vi "Read Users file (popup).vi"(0 "file path (use dialog)":path, 11 "error in (no error)":errorcluster) -> (15 "error out":errorcluster)   [LabVIEW 2012]
doc: "Demo for Type Sensitive Popup\n\nType Sensitive Popup \nCopyright © 2007, J. David Saunders\nAll rights reserved."
uses:
  Desktop/PFC/TypeSensitivePopup_V1_0_1/SubVIs/TSPopup.Popup Cluster.ctl
  Desktop/PFC/TypeSensitivePopup_V1_0_1/SubVIs/TSPopup.Grid.Cell Info.ctl
  Desktop/PFC/TypeSensitivePopup_V1_0_1/SubVIs/TSPopup.Data Type.ctl
  Desktop/PFC/TypeSensitivePopup_V1_0_1/SubVIs/TSPopup.Popup Call Parameters.ctl
  type def/Hyde&Show.ctl
panel:
  out "Info accounts 2":bool
  out "Info pass not secure":bool
  out "Info Dupliclate user":bool
  out "Duplicate user":string[][](table)
  out "Password not secure":string[][](table)
  out "Info accounts":bool
  in  "Cuenta":bool
  in  "Clave":bool
  in  "Name":bool
  in  "Reload":bool
  in  "Save":bool
  in  "Check changes":bool
  in  "Delete":bool
  in  "Show Popup (type only)":T1
  in  "Popups":T3 {"Boolean" items=["False", "True"]; "Ring" items=["None", "User", "Admin"]}
  in  "Cell Info (type only)":T4
  in  "Cancel":bool
  in  "?":string[][](table)
  # "Type Sensitive\nPopup"
  # "Boolean Colors"
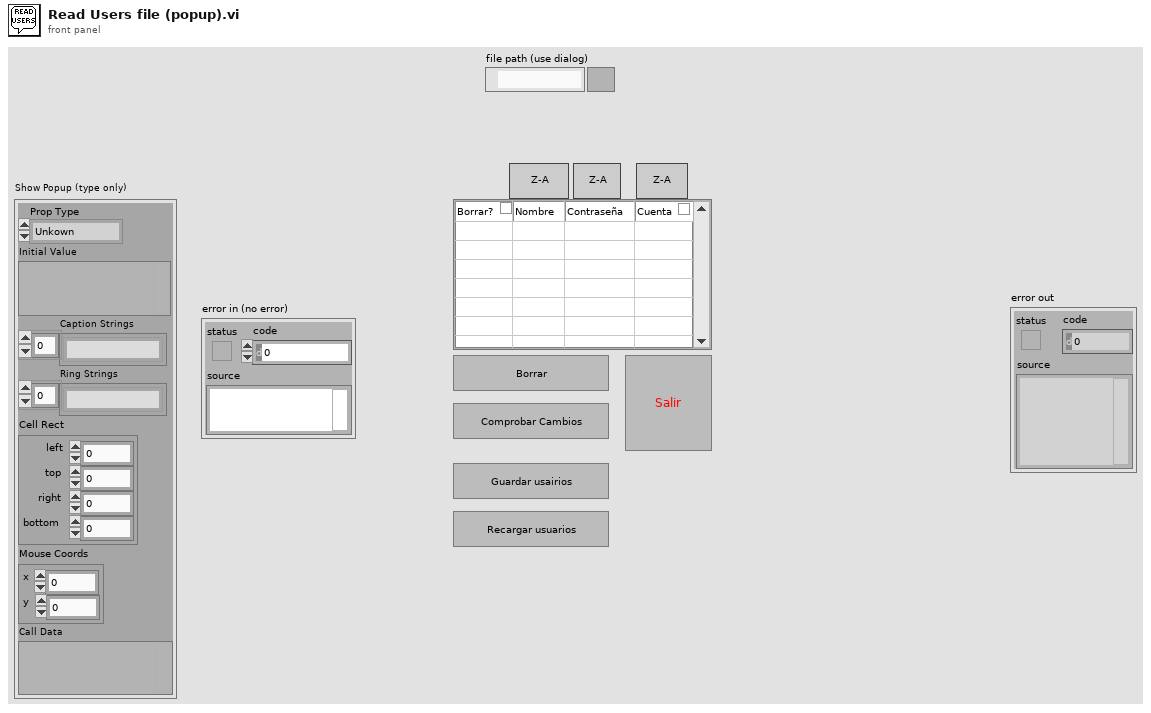
[diagram p1: front panel]
types:
  T1 = typedef "TSPopup.Popup Call Parameters.ctl" = cluster{"Prop Type":T2, "Initial Value":variant, "Caption Strings":string[], "Ring Strings":string[], "Cell Rect":cluster{"left":i16, "top":i16, "right":i16, "bottom":i16}, "Mouse Coords":cluster{"x":i16, "y":i16}, "Call Data":variant}
  T2 = typedef "TSPopup.Data Type.ctl" = enum16{"Unkown", "NO POPUP", "String", "Integer", "Float", "Color", "Boolean", "Ring", "Captioned String", "Captioned Integer", "Button Color", "2 Int Cluster", "4 Int Cluster"}
  T3 = typedef "TSPopup.Popup Cluster.ctl" = cluster{"Unknown":bool, "Unknown 2":bool, "String":string, "Integer":i32, "Float":dbl, "Color":u32, "Boolean":u32, "Ring":u32, "Captioned String":cluster{"String":string, "OK":bool, "Cancel":bool}, "Captioned Integer":cluster{"First":i32, "OK":bool, "Cancel":bool}, "Boolean Colors":cluster{"False":cluster{"FG":u32, "BG":u32}, "True":cluster{"FG":u32, "BG":u32}, "T  to  F":cluster{"FG":u32, "BG":u32}, "F  to  T":cluster{"FG":u32, "BG":u32}, "OK":bool, "Cancel":bool}, "2-Int Cluster":cluster{"First":i32, "Second":i32, "OK":bool, "Cancel":bool}, "4-Int Cluster":cluster{"First":i32, "Second":i32, "Third":i32, "Fourth":i32, "OK":bool, "Cancel":bool}}
  T4 = typedef "TSPopup.Grid.Cell Info.ctl" = cluster{"Tag":string, "Row":i32, "Column":i32, "In Symbol?":bool, "In Data?":bool, "Cell String":string, "Ctl Refnum":refnum<vi>, "Prop Type":T2, "Ring Strings":string[]}
  T5 = typedef "User_Data_Cluster.ctl" = cluster{"Usuario":string, "Password":string, "Account type":T6, "Time Stamp":timestamp}
  T6 = typedef "User Accounts.ctl" = enum16{"None", "User", "Admin"}
  T7 = typedef "LVPoint32TypeDef.ctl" = cluster{"Horizontal":i32, "Vertical":i32}
  T8 = typedef "Hyde&Show.ctl" = enum8{"Enabled", "Disabled", " Grayed Out", "Hide"}
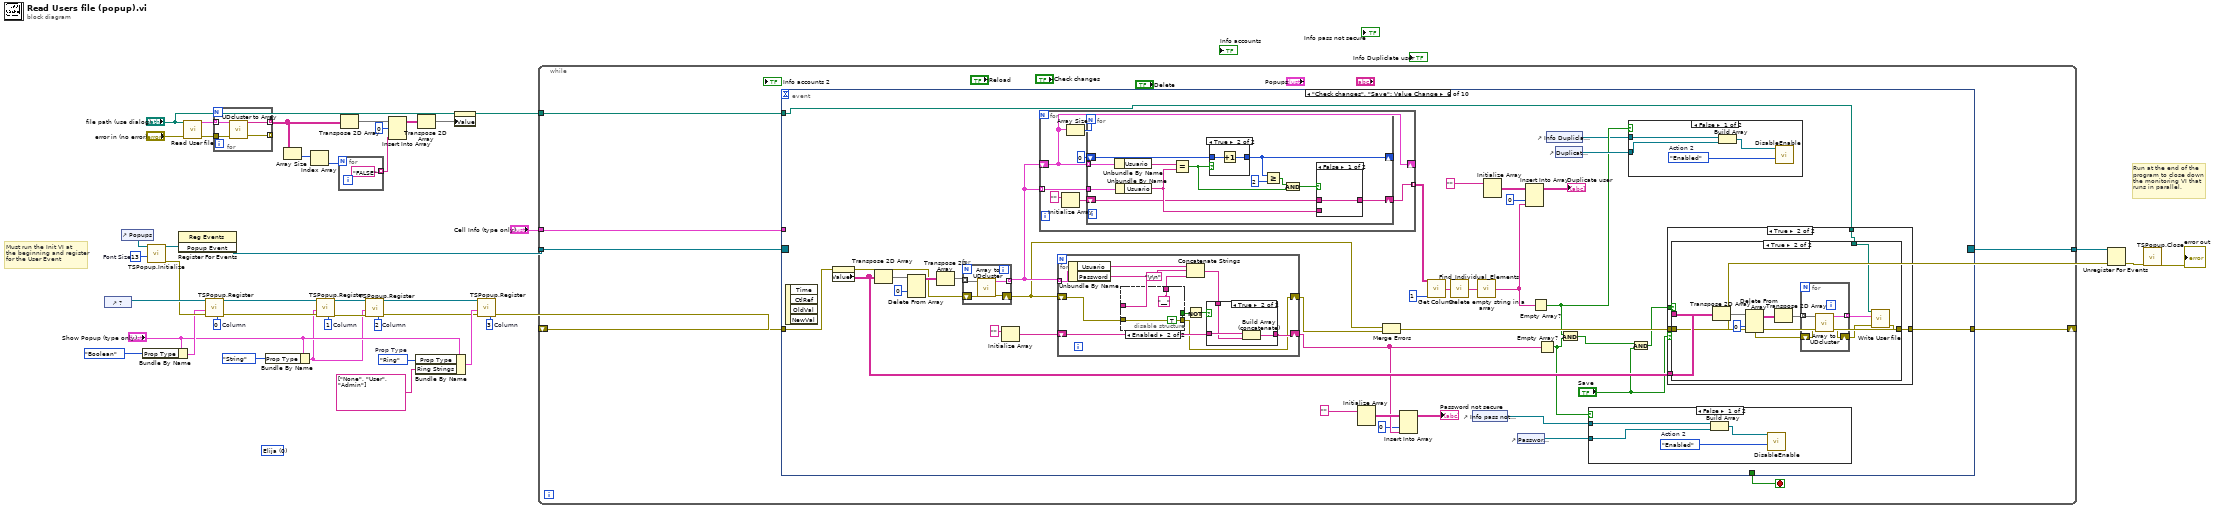
[diagram p0: block diagram]
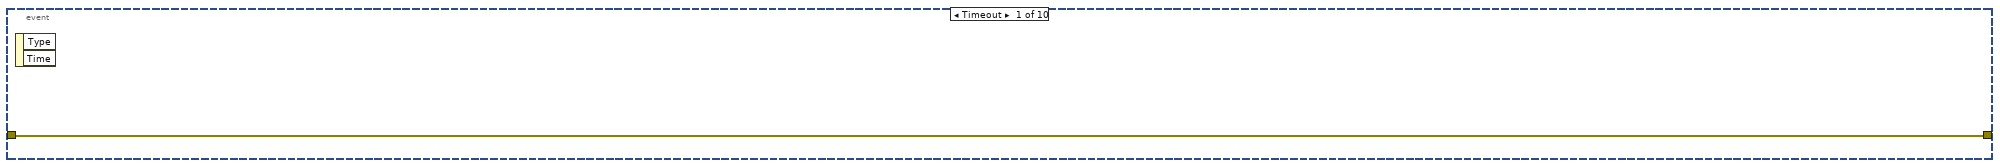
[diagram p2: hidden frame]
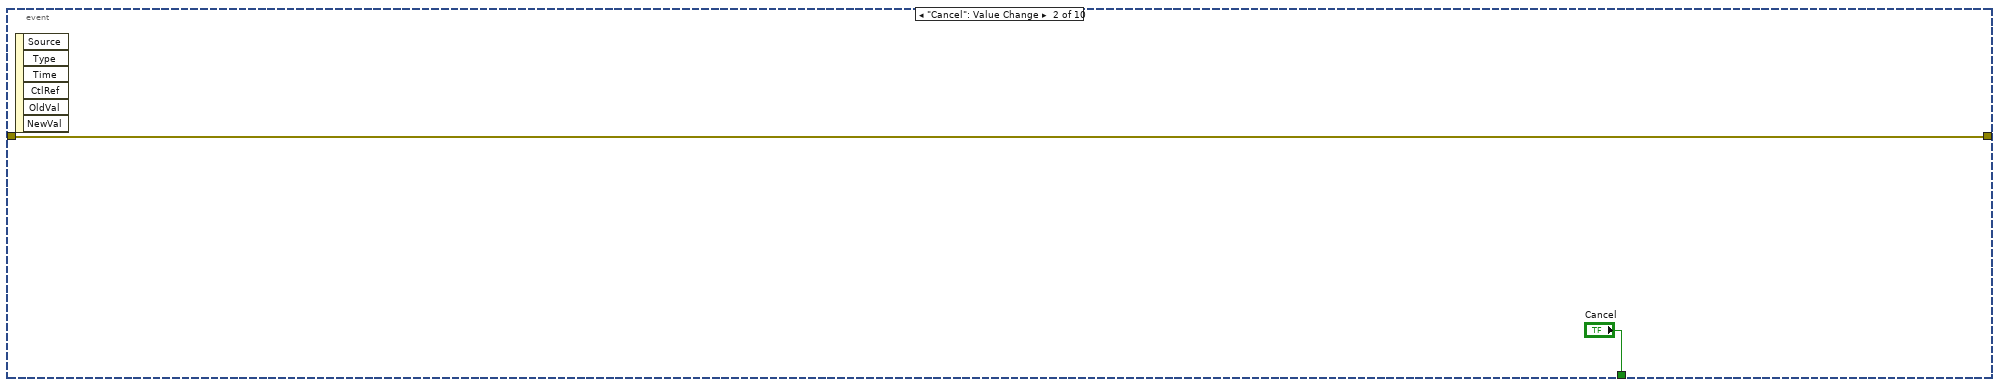
[diagram p3: hidden frame]
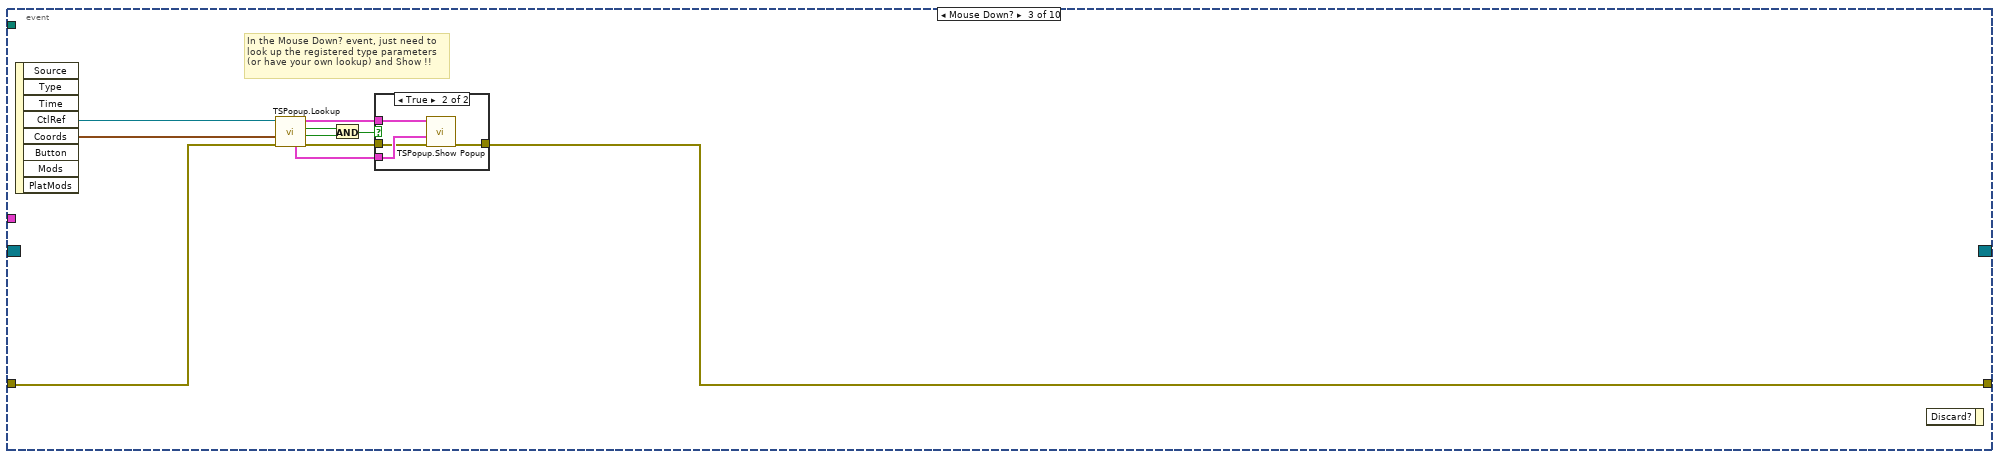
[diagram p4: hidden frame]
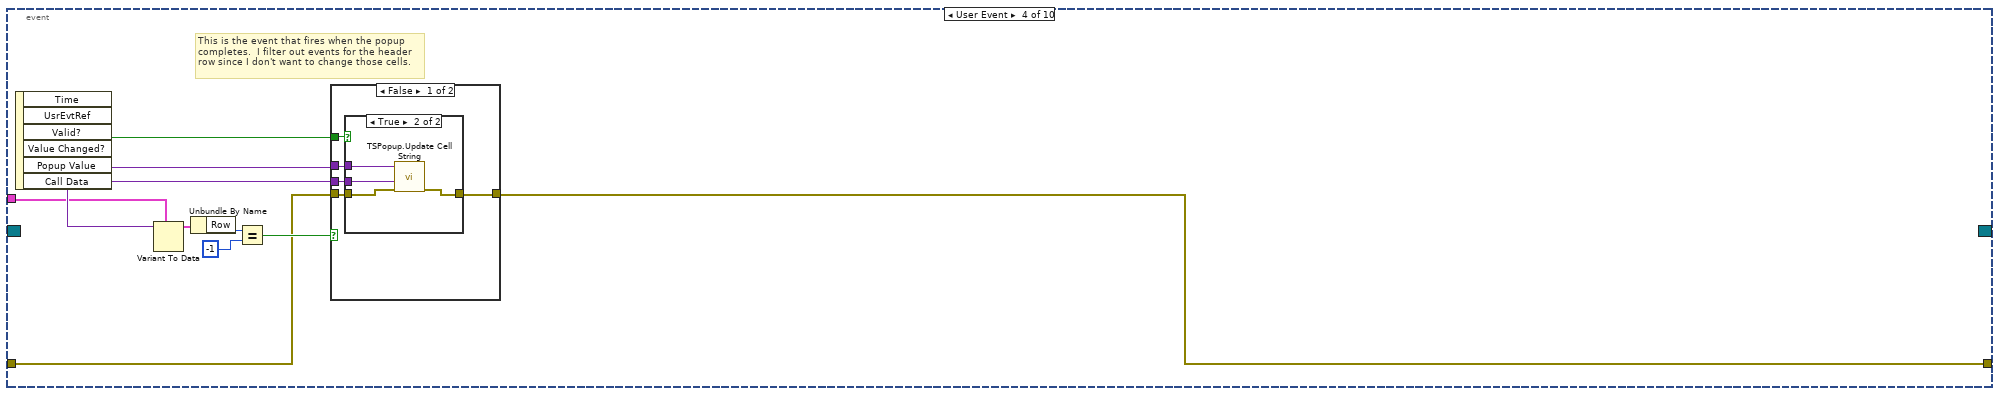
[diagram p6: hidden frame]
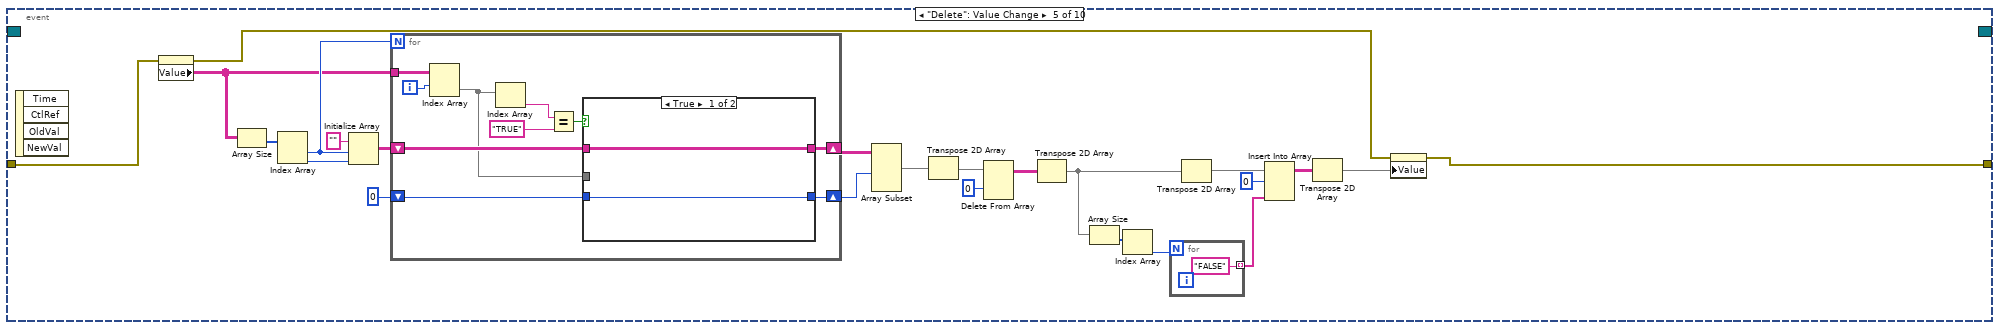
[diagram p9: hidden frame]
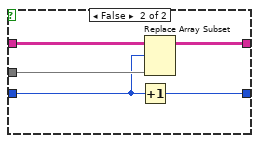
[diagram p10: hidden frame]
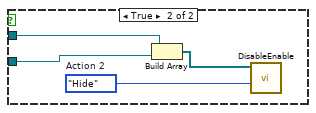
[diagram p11: hidden frame]
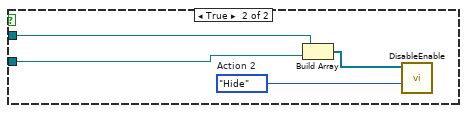
[diagram p12: hidden frame]
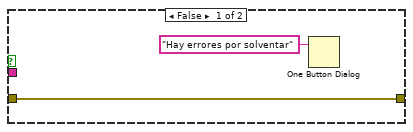
[diagram p14: hidden frame]
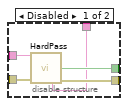
[diagram p15: hidden frame]
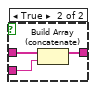
[diagram p17: hidden frame]
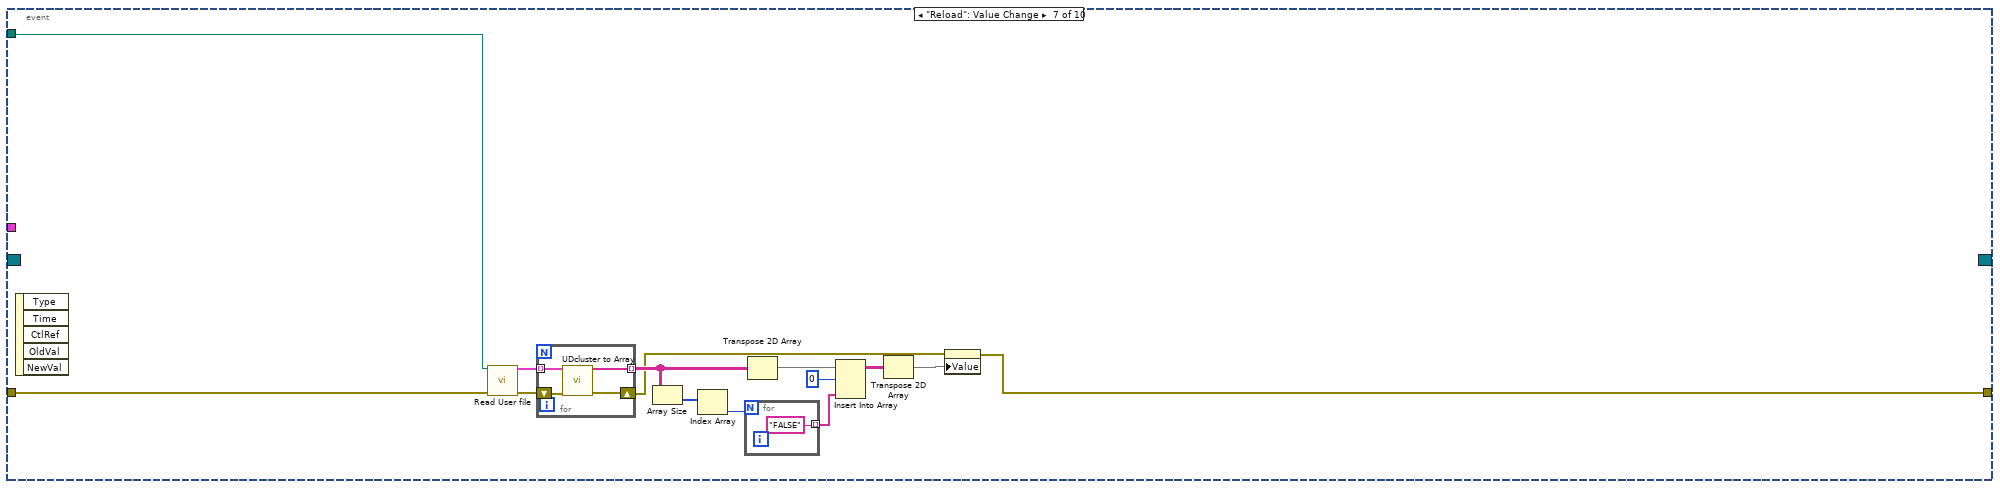
[diagram p19: hidden frame]
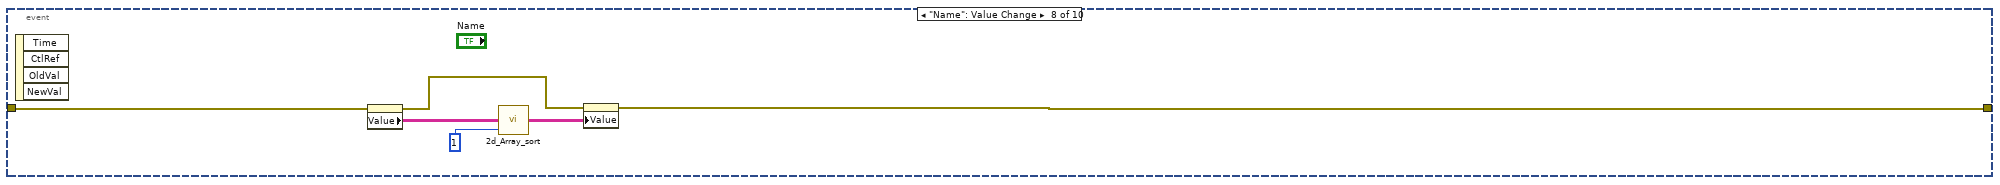
[diagram p20: hidden frame]
diagram:
  (unwired) u16 0 items=["Elija", "Comprobar cambios", "Recargar usuarios", "Borrar usuarios"] ("Ring")
  w17 = 2  # Column
  w30 = 0  # Column
  w31 = 1  # Column
  w33 = 3  # Column
  w35 = TSPopup.Data_Type."Ring"  # Prop Type
  w41 = u32 13  # Font Size
  # "Run at the end of the\nprogram to close down\nthe monitoring VI that\nruns in parallel."
  # "Must run the Init VI at\nthe beginning and register\nfor the User Event"
  n1 = control-ref of="?"() -> (w26:refnum<vi>)
  n2 = control-ref of="Popups"() -> (w42:refnum<vi>)
  n3 = Bundle By Name(cluster="Show Popup (type only)", "Prop Type"=TSPopup.Data_Type."Boolean") -> (w24:T1)
  n4 = call "TSPopup.Initialize.vi"("Font Size"=w41, "Popup Cluster Ref"=w42) -> ("error out"=w25:errorcluster, "Popup Event"=w40:refnum<user-event>)  [unwired: 8 in]
  n5 = register-events(w40) -> (reference out=w39:refnum<event-registration>)  [unwired: 2 in, 1 out]
  n6 = call "Read User file.vi"("file path (use dialog)"="file path (use dialog)", "error in"="error in (no error)") -> ("Array"=w4:T5[], "error out"=w23:errorcluster)  [unwired: 12 in]
  n7 = call "TSPopup.Register.vi"("Col (unwired = all columns)"=w30, "error in (no error)"=w25, "Parameters"=w24, "Ctl Refnum"=w26) -> ("error out"=w28:errorcluster, "dup ref out"=w29:refnum<vi>)  [unwired: 6 in]
  n8 = for {
    tunnel: [w46] -> w5 mode=indexing
    tunnel: w4 -> [w45] mode=indexing
    tunnel: w23 -> [w44]
    tunnel: [w43] -> _ mode=indexing
    n9 = call "UDcluster to Array.vi"("User-data cluster"=w45, "error in (no error)"=w44) -> ("UD array"=w46:string[], "error out"=w43:errorcluster)  [unwired: 12 in]
  }
  n10 = Bundle By Name(cluster="Show Popup (type only)", "Prop Type"=TSPopup.Data_Type."String") -> (w9:T1)
  n11 = Array Size(array=w5) -> (size(s)=w7:i32[])
  n12 = Index Array(array=w7) -> (element=w6:i32)  [unwired: 1 in]
  n13 = call "TSPopup.Register.vi"("Col (unwired = all columns)"=w31, "error in (no error)"=w28, "Parameters"=w9, "Ctl Refnum"=w29) -> ("error out"=w14:errorcluster, "dup ref out"=w10:refnum<vi>)  [unwired: 6 in]
  n14 = for {
    N: w6 -> [_]
    tunnel: ["FALSE"] -> w8 mode=indexing
  }
  n15 = Transpose 2D Array(2D array=w5) -> (transposed array=w20:string[][])
  n16 = call "TSPopup.Register.vi"("Col (unwired = all columns)"=w17, "error in (no error)"=w14, "Parameters"=w9, "Ctl Refnum"=w10) -> ("error out"=w15:errorcluster, "dup ref out"=w16:refnum<vi>)  [unwired: 6 in]
  n17 = Insert Into Array(array=w20, index (row)=0, new element=w8) -> (w21:string[][])  [unwired: 1 in]
  n18 = Bundle By Name(cluster="Show Popup (type only)", "Prop Type"=w35, "Ring Strings"=string[] ["None", "User", "Admin"]) -> (w34:T1)
  n19 = Transpose 2D Array(2D array=w21) -> (transposed array=w18:string[][])
  n20 = property class="Tbl (strict)"("Value"=w18) -> ()  [unwired: 2 in, 2 out]
  n21 = call "TSPopup.Register.vi"("Col (unwired = all columns)"=w33, "error in (no error)"=w15, "Parameters"=w34, "Ctl Refnum"=w16) -> ("error out"=w11:errorcluster)  [unwired: 6 in, 1 out]
  n22 = while {
    tunnel: w39 -> [w54]
    tunnel: [w53] -> w38
    tunnel: "Cell Info (type only)" -> [w52]
    tunnel: "file path (use dialog)" -> [w50]
    shift-right: [w49] -> w2
    shift-left: w11 -> [w51]
    stop <- w48 stop-if-true
    n23 = event shown="[5] \"Check changes\", \"Save\": Value Change" {
      selector: w54 -> [_ _ _ _ _ _ _ _ _ _]
      dyn-events: [_ _ _ _ _ _ _ _ _ _] -> w53
      timeout: _ -> [_ _ _ _ _ _ _ _ _ _]
      tunnel: w52 -> [_ _ _ w75 _ _ _ _ _ _]
      tunnel: w51 -> [w55 w57 w59 w74 w96 w166 w270 w288 _ _]
      tunnel: w50 -> [_ _ _ _ _ w154 w269 _ _ _]
      tunnel: [w55 w57 w58 w73 w94 w160 w266 w287 _ _] -> w49
      tunnel: [_ "Cancel" _ _ _ _ _ _ _ _] -> w48
      event Timeout {
        n24 = event-data() -> ()  [unwired: 1 in, 2 out]
      }
      event "Cancel": Value Change {
        n25 = event-data() -> ()  [unwired: 1 in, 6 out]
      }
      event Mouse Down? {
        # "In the Mouse Down? event, just need to\nlook up the registered type parameters\n(or have your own lookup) and Show !!"
        n26 = event-data() -> ("CtlRef"=w67:refnum<vi>, "Coords"=w66:T7)  [unwired: 1 in, 6 out]
        n27 = call "TSPopup.Lookup.vi"("error in (no error)"=w59, "Point"=w66, "Ctl Refnum"=w67) -> ("error out"=w60:errorcluster, "In Bounds?"=w64:bool, "Found"=w65:bool, "Popup Parameters"=w62:T1, "Cell Info (Call data)"=w61:T4)  [unwired: 4 in]
        n28 = And(x=w65, y=w64) -> (x .and. y?=w63:bool)
        n29 = case shown="True" w63 {
          tunnel: w62 -> [_ w72]
          tunnel: w61 -> [_ w71]
          tunnel: w60 -> [w68 w70]
          tunnel: [w68 w69] -> w58
          frame False {
          }
          frame True {
            n30 = call "TSPopup.Show Popup.vi"("error in (no error)"=w70, "Call Data (ignore if empty)"=w71, "Popup Parameters"=w72) -> ("error out"=w69:errorcluster)  [unwired: 8 in]
          }
        }
        n31 = event-data() -> ()  [unwired: 2 in, 1 out]
      }
      event User Event {
        # "This is the event that fires when the popup\ncompletes.  I filter out events for the header\nrow since I don't want to change those cells."
        n32 = event-data() -> ("Valid?"=w82:bool, "Popup Value"=w81:variant, "Call Data"=w80:variant)  [unwired: 1 in, 3 out]
        n33 = Variant To Data(type=w75, Variant=w80) -> (data=w79:T4)  [unwired: 1 in, 1 out]
        n34 = Unbundle By Name(w79) -> ("Row"=w78:i32)
        n35 = Equal?(x=w78, y=-1) -> (x = y?=w76:bool)
        n36 = case shown="False" w76 {
          tunnel: w82 -> [w87 _]
          tunnel: w81 -> [w86 _]
          tunnel: w80 -> [w85 _]
          tunnel: w74 -> [w84 w93]
          tunnel: [w83 w93] -> w73
          frame False {
            n37 = case shown="True" w87 {
              tunnel: w86 -> [_ w91]
              tunnel: w85 -> [_ w92]
              tunnel: w84 -> [w88 w90]
              tunnel: [w88 w89] -> w83
              frame False {
              }
              frame True {
                n38 = call "TSPopup.Update Cell String.vi"("error in (no error)"=w90, "Call Data (must be Cell Info cluster)"=w92, "Popup Value"=w91) -> ("error out"=w89:errorcluster)  [unwired: 8 in]
              }
            }
          }
          frame True {
          }
        }
      }
      event "Delete": Value Change {
        n39 = event-data() -> ()  [unwired: 1 in, 4 out]
        n40 = property class="Tbl (strict)"(error in=w96) -> (error out=w95:errorcluster, "Value"=w105:string[][])  [unwired: 1 in, 1 out]
        n41 = Array Size(array=w105) -> (size(s)=w115:i32[])
        n42 = Index Array(array=w115) -> (element #1=w116:i32, element #2=w117:i32)  [unwired: 2 in]
        n43 = Initialize Array("", w116, w117) -> (w111:string[][])
        n44 = for {
          N: w116 -> [_]
          tunnel: w105 -> [w123]
          shift-right: [w126] -> w114
          shift-left: 0 -> [w125]
          shift-right: [w124] -> w113
          shift-left: w111 -> [w127]
          i -> [w128]
          n45 = Index Array(array=w123, index (row)=w128) -> (element=w122:string[])  [unwired: 1 in]
          n46 = Index Array(array=w122) -> (element=w120:string)  [unwired: 1 in]
          n47 = Equal?(x=w120, y="TRUE") -> (x = y?=w121:bool)
          n48 = case shown="True" w121 {
            tunnel: w127 -> [w130 w135]
            tunnel: [w129 w134] -> w126
            tunnel: w125 -> [w129 w131]
            tunnel: [w130 w133] -> w124
            tunnel: w122 -> [_ w132]
            frame True {
            }
            frame False {
              n49 = Increment(x=w131) -> (x+1=w134:i32)
              n50 = Replace Array Subset(array=w135, new element=w132, index (row)=w131) -> (w133:string[][])  [unwired: 1 in]
            }
          }
        }
        n51 = Array Subset(array=w113, length (row)=w114) -> (w106:string[][])  [unwired: 3 in]
        n52 = Transpose 2D Array(2D array=w106) -> (transposed array=w109:string[][])
        n53 = Delete From Array(array=w109, index (row)=0) -> (array with subset deleted=w107:string[][])  [unwired: 2 in, 1 out]
        n54 = Transpose 2D Array(2D array=w107) -> (transposed array=w97:string[][])
        n55 = Array Size(array=w97) -> (size(s)=w100:i32[])
        n56 = Index Array(array=w100) -> (element=w99:i32)  [unwired: 1 in]
        n57 = for {
          N: w99 -> [_]
          tunnel: ["FALSE"] -> w101 mode=indexing
        }
        n58 = Transpose 2D Array(2D array=w97) -> (transposed array=w103:string[][])
        n59 = Insert Into Array(array=w103, index (row)=0, new element=w101) -> (w104:string[][])  [unwired: 1 in]
        n60 = Transpose 2D Array(2D array=w104) -> (transposed array=w98:string[][])
        n61 = property class="Tbl (strict)"(error in=w95, "Value"=w98) -> (error out=w94:errorcluster)  [unwired: 1 in, 1 out]
      }
      event "Check changes", "Save": Value Change {
        n62 = event-data() -> ()  [unwired: 1 in, 4 out]
        n63 = property class="Tbl (strict)"(error in=w166) -> (error out=w165:errorcluster, "Value"=w161:string[][])  [unwired: 1 in, 1 out]
        n64 = Transpose 2D Array(2D array=w161) -> (transposed array=w173:string[][])
        n65 = Delete From Array(array=w173, index (row)=0) -> (array with subset deleted=w171:string[][])  [unwired: 2 in, 1 out]
        n66 = Transpose 2D Array(2D array=w171) -> (transposed array=w169:string[][])
        n67 = for {
          tunnel: [w265] -> w170 mode=indexing
          tunnel: w169 -> [w264] mode=indexing
          shift-right: [w263] -> w143
          shift-left: w165 -> [w262]
          n68 = call "Array to UDcluster.vi"("UD array"=w264, "error in (no error)"=w262) -> ("User-data cluster out"=w265:T5, "error out"=w263:errorcluster)  [unwired: 12 in]
        }
        n69 = Initialize Array("") -> (w167:string[])  [unwired: 1 in]
        n70 = for {
          shift-right: [w239] -> _
          shift-left: w170 -> [w239]
          tunnel: w170 -> [w242] mode=indexing
          tunnel: [w236] -> w164 mode=indexing
          n71 = Initialize Array("") -> (w237:string[])  [unwired: 1 in]
          n72 = Array Size(array=w239) -> (size(s)=w241:i32)
          n73 = for {
            N: w241 -> [_]
            tunnel: w242 -> [w254]
            tunnel: w239 -> [w253] mode=indexing
            shift-right: [w246] -> _
            shift-left: 0 -> [w251]
            shift-right: [w244] -> w236
            shift-left: w237 -> [w243]
            n74 = Unbundle By Name(w253) -> ("Usuario"=w252:string)
            n75 = Unbundle By Name(w254) -> ("Usuario"=w245:string)
            n76 = Equal?(x=w252, y=w245) -> (x = y?=w247:bool)
            n77 = case shown="True" w247 {
              tunnel: w251 -> [w259 w261]
              tunnel: [w259 w260] -> w246
              frame False {
              }
              frame True {
                n78 = Increment(x=w261) -> (x+1=w260:i32)
              }
            }
            n79 = Greater Or Equal?(x=w246, y=2) -> (x >= y?=w250:bool)
            n80 = And(x=w250, y=w247) -> (x .and. y?=w248:bool)
            n81 = case shown="False" w248 {
              tunnel: w243 -> [w255 w257]
              tunnel: w245 -> [_ w256]
              tunnel: [w255 w258] -> w244
              frame False {
              }
              frame True {
                n82 = Build Array (concatenate)(w257, w256) -> (w258:string[])
              }
            }
          }
        }
        n83 = for {
          tunnel: w170 -> [w223] mode=indexing
          shift-right: [w221] -> w151
          shift-left: w167 -> [w220]
          shift-right: [w216] -> w142
          shift-left: w143 -> [w217]
          n84 = Unbundle By Name(w223) -> ("Usuario"=w215:string, "Password"=w222:string)
          n85 = disable-structure shown="Enabled" {
            disable-tunnel: w222 -> [w228 _]
            disable-tunnel: w217 -> [w227 w231]
            disable-tunnel: [w226 w231] -> w216
            disable-tunnel: [w225 TRUE ("Hard enough?")] -> w218
            disable-tunnel: [w224 "__" ("What is missed")] -> w214
            frame Disabled {
              n86 = call "HardPass.vi"("Password"=w228, "error in (no error)"=w227) -> ("Hard enough?"=w225:bool, "What is missed"=w224:string, "error out"=w226:errorcluster)  [unwired: 10 in, 1 out]
            }
            frame Enabled {
            }
          }
          n87 = Concatenate Strings(w215, "\r\n", w214) -> (w212:string)
          n88 = Not(x=w218) -> (.not. x?=w219:bool)
          n89 = case shown="True" w219 {
            tunnel: w212 -> [_ w234]
            tunnel: w220 -> [w232 w235]
            tunnel: [w232 w233] -> w221
            frame False {
            }
            frame True {
              n90 = Build Array (concatenate)(w235, w234) -> (w233:string[])
            }
          }
        }
        n91 = Initialize Array("") -> (w152:string[][])  [unwired: 2 in]
        n92 = Merge Errors(w143, w142) -> (w159:errorcluster)
        n93 = Insert Into Array(array=w152, index (col)=0 ("disabled index (col)"), new element=w151) -> (→"Password not secure":string[][])  [unwired: 1 in]
        n94 = call "Get Column.vi"("2D Array Input"=w164, "Column Number"=1) -> ("1D Column Array"=w162:string[])  [unwired: 13 in]
        n95 = call "Find_Individual_Elements.vi"("Array In"=w162) -> ("Array Out"=w158:string[])  [unwired: 14 in]
        n96 = control-ref of="Info pass not secure"() -> (w137:refnum<vi>)
        n97 = call "Delete empty string in a array.vi"("Array in"=w158) -> ("Array out"=w144:string[])  [unwired: 14 in]
        n98 = Initialize Array("") -> (w147:string[][])  [unwired: 2 in]
        n99 = control-ref of="Password not secure"() -> (w140:refnum<vi>)
        n100 = Insert Into Array(array=w147, index (col)=0 ("disabled index (col)"), new element=w144) -> (→"Duplicate user":string[][])  [unwired: 1 in]
        n101 = Empty Array?(array=w144) -> (empty?=w138:bool)
        n102 = Empty Array?(array=w151) -> (empty?=w141:bool)
        n103 = control-ref of="Info Dupliclate user"() -> (w136:refnum<vi>)
        n104 = control-ref of="Duplicate user"() -> (w139:refnum<vi>)
        n105 = And(x=w138, y=w141) -> (x .and. y?=w157:bool)
        n106 = case shown="False" w141 {
          tunnel: w137 -> [w183 w187]
          tunnel: w140 -> [w182 w186]
          frame False {
            w185 = Hyde&Show."Enabled"  # Action 2
            n107 = Build Array(w183, w182) -> (w184:refnum<vi>[])
            n108 = call "DisableEnable.vi"("Action 2"=w185, "Array of Control References"=w184) -> ()  [unwired: 9 in, 1 out]
          }
          frame True {
            w189 = Hyde&Show."Hide"  # Action 2
            n109 = Build Array(w187, w186) -> (w188:refnum<vi>[])
            n110 = call "DisableEnable.vi"("Action 2"=w189, "Array of Control References"=w188) -> ()  [unwired: 9 in, 1 out]
          }
        }
        n111 = case shown="False" w138 {
          tunnel: w136 -> [w175 w179]
          tunnel: w139 -> [w174 w178]
          frame False {
            w177 = Hyde&Show."Enabled"  # Action 2
            n112 = Build Array(w175, w174) -> (w176:refnum<vi>[])
            n113 = call "DisableEnable.vi"("Action 2"=w177, "Array of Control References"=w176) -> ()  [unwired: 9 in, 1 out]
          }
          frame True {
            w181 = Hyde&Show."Hide"  # Action 2
            n114 = Build Array(w179, w178) -> (w180:refnum<vi>[])
            n115 = call "DisableEnable.vi"("Action 2"=w181, "Array of Control References"=w180) -> ()  [unwired: 9 in, 1 out]
          }
        }
        n116 = And(x=w157, y="Save") -> (x .and. y?=w155:bool)
        n117 = case shown="True" "Save" {
          tunnel: [w190 w195] -> w160
          tunnel: w161 -> [_ w194]
          tunnel: w159 -> [w190 w193]
          tunnel: w155 -> [_ w192]
          tunnel: w154 -> [_ w191]
          frame False {
          }
          frame True {
            n118 = case shown="True" w192 {
              tunnel: [w197 w201] -> w195
              tunnel: w194 -> [_ w200]
              tunnel: w193 -> [w197 w199]
              tunnel: w191 -> [_ w198]
              frame False {
                n119 = One Button Dialog(message="Hay errores por solventar") -> ()  [unwired: 1 in, 1 out]
              }
              frame True {
                n120 = Transpose 2D Array(2D array=w200) -> (transposed array=w207:string[][])
                n121 = Delete From Array(array=w207, index (row)=0) -> (array with subset deleted=w205:string[][])  [unwired: 2 in, 1 out]
                n122 = Transpose 2D Array(2D array=w205) -> (transposed array=w204:string[][])
                n123 = for {
                  tunnel: [w211] -> w203 mode=indexing
                  tunnel: w204 -> [w210] mode=indexing
                  shift-right: [w208] -> w202
                  shift-left: w199 -> [w209]
                  n124 = call "Array to UDcluster.vi"("UD array"=w210, "error in (no error)"=w209) -> ("User-data cluster out"=w211:T5, "error out"=w208:errorcluster)  [unwired: 12 in]
                }
                n125 = call "Write User file.vi"("error in"=w202, "Array"=w203, "file path (use dialog)"=w198) -> ("error out"=w201:errorcluster)  [unwired: 7 in, 1 out]
              }
            }
          }
        }
      }
      event "Reload": Value Change {
        n126 = event-data() -> ()  [unwired: 1 in, 5 out]
        n127 = call "Read User file.vi"("file path (use dialog)"=w269, "error in"=w270) -> ("Array"=w271:T5[], "error out"=w268:errorcluster)  [unwired: 12 in]
        n128 = for {
          tunnel: [w284] -> w272 mode=indexing
          tunnel: w271 -> [w283] mode=indexing
          shift-right: [w282] -> w267
          shift-left: w268 -> [w281]
          n129 = call "UDcluster to Array.vi"("User-data cluster"=w283, "error in (no error)"=w281) -> ("UD array"=w284:string[], "error out"=w282:errorcluster)  [unwired: 12 in]
        }
        n130 = Array Size(array=w272) -> (size(s)=w274:i32[])
        n131 = Index Array(array=w274) -> (element=w273:i32)  [unwired: 1 in]
        n132 = for {
          N: w273 -> [_]
          tunnel: ["FALSE"] -> w275 mode=indexing
        }
        n133 = Transpose 2D Array(2D array=w272) -> (transposed array=w278:string[][])
        n134 = Insert Into Array(array=w278, index (row)=0, new element=w275) -> (w279:string[][])  [unwired: 1 in]
        n135 = Transpose 2D Array(2D array=w279) -> (transposed array=w276:string[][])
        n136 = property class="Tbl (strict)"(error in=w267, "Value"=w276) -> (error out=w266:errorcluster)  [unwired: 1 in, 1 out]
      }
      event "Name": Value Change {
        n137 = event-data() -> ()  [unwired: 1 in, 4 out]
        n138 = property class="Tbl (strict)"(error in=w288) -> (error out=w289:errorcluster, "Value"=w290:string[][])  [unwired: 1 in, 1 out]
        n139 = call "2d_Array_sort.vi"("Column to Sort on"=u16 1, "2D Input Array"=w290) -> ("2D Ouput Array"=w285:string[][])  [unwired: 1 in]
        n140 = property class="Tbl (strict)"(error in=w289, "Value"=w285) -> (error out=w287:errorcluster)  [unwired: 1 in, 1 out]
      }
      event "Clave": Value Change {
        n141 = event-data() -> ()  [unwired: 1 in, 4 out]
        n142 = property class="Tbl (strict)"() -> (error out=w294:errorcluster, "Value"=w295:string[][])  [unwired: 2 in, 1 out]
        n143 = call "2d_Array_sort.vi"("Column to Sort on"=u16 1, "2D Input Array"=w295, "Sort numerically"="Clave") -> ("2D Ouput Array"=w292:string[][])
        n144 = property class="Tbl (strict)"(error in=w294, "Value"=w292) -> ()  [unwired: 1 in, 2 out]
      }
      event "Cuenta": Value Change {
        n145 = event-data() -> ()  [unwired: 1 in, 4 out]
        n146 = property class="Tbl (strict)"() -> (error out=w299:errorcluster, "Value"=w300:string[][])  [unwired: 2 in, 1 out]
        n147 = call "2d_Array_sort.vi"("Column to Sort on"=u16 1, "2D Input Array"=w300, "Sort numerically"="Cuenta") -> ("2D Ouput Array"=w297:string[][])
        n148 = property class="Tbl (strict)"(error in=w299, "Value"=w297) -> ()  [unwired: 1 in, 2 out]
      }
    }
  }
  n149 = Unregister For Events(event registration refnum=w38, error in=w2) -> (error out=w37:errorcluster)
  n150 = call "TSPopup.Close.vi"("error in (no error)"=w37) -> ("error out"=→"error out":errorcluster)  [unwired: 10 in]
